vi "Cycling_No_DAQ_Tasks.vi"() -> ()   [LabVIEW 2020]
uses:
  IT-M3400/IT-M3400.lvlib
panel:
  in  "Number of Cycles":i32
  in  "Charge filepath":path
  in  "Discharge filepath":path
  in  "Batteryname":string
  in  "Starting Cycle":i32
  out "PS error out":errorcluster
  out "PS Visa Out":refnum<visa-resource-name>
  in  "Wait time":dbl
  in  "Discharge Current Setpoint":dbl format="%#.6g"
  in  "Charge Current Setpoint":dbl format="%#.6g"
  in  "Battery Type":enum16{"30Q", "40T"}(ring)
  in  "PS type":enum16{"NHR", "ITECH"}(ring)
  in  "PS error in":errorcluster caption="PS error in (no error)"
  in  "PS VISA in":refnum<visa-resource-name>
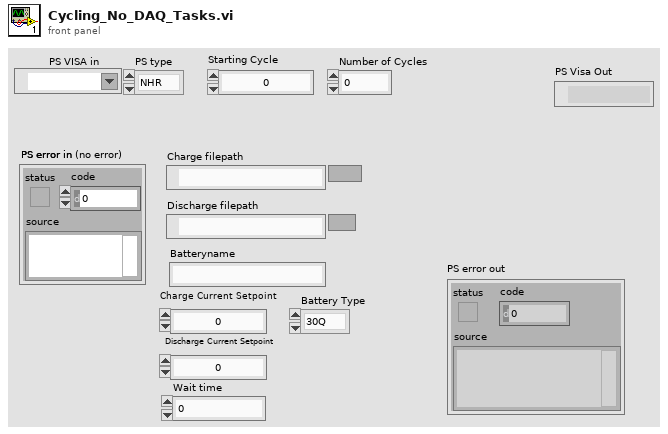
[diagram p1: front panel]
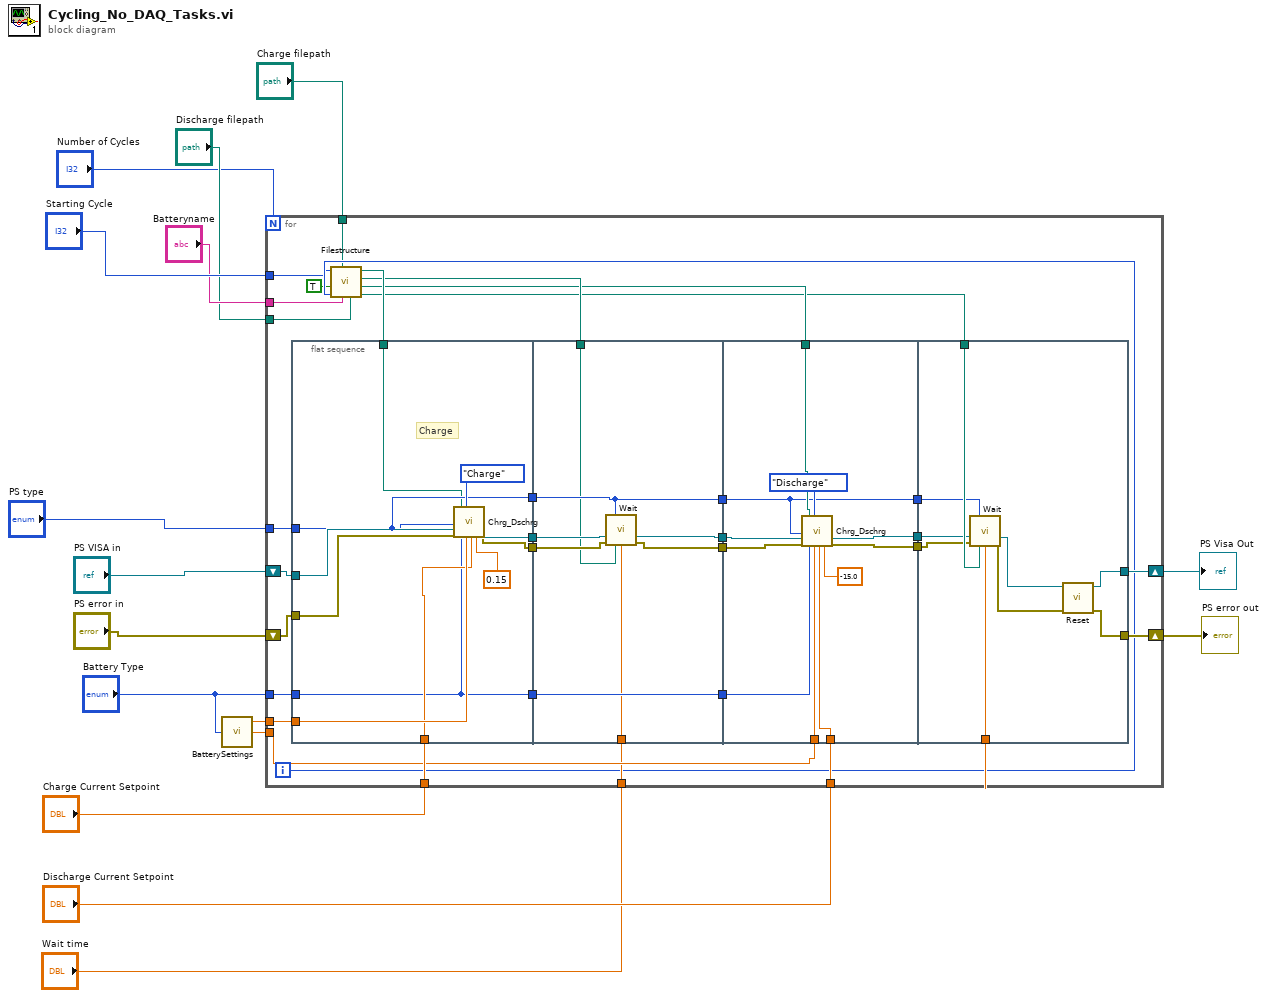
[diagram p0: block diagram]
diagram:
  n1 = call "BatterySettings.vi"("Battery Type"="Battery Type") -> ("Min Voltage (V)"=w10:dbl, "Max Voltage (V)"=w13:dbl)  [unwired: 2 in, 1 out]
  n2 = for {
    N: "Number of Cycles" -> [_]
    tunnel: "PS type" -> [w37]
    tunnel: w13 -> [w34]
    tunnel: "Battery Type" -> [w33]
    tunnel: "Charge Current Setpoint" -> [w32]
    tunnel: w10 -> [w31]
    tunnel: "Discharge Current Setpoint" -> [w30]
    tunnel: "Wait time" -> [w25]
    shift-right: [w23] -> w6
    shift-left: "PS VISA in" -> [w36]
    shift-right: [w24] -> w7
    shift-left: "PS error in" -> [w35]
    tunnel: "Starting Cycle" -> [w21]
    tunnel: "Batteryname" -> [w19]
    tunnel: "Discharge filepath" -> [w18]
    tunnel: "Charge filepath" -> [w17]
    i -> [w22]
    n3 = flat-sequence {
      tunnel: w37 -> [w51]
      tunnel: w36 -> [w59]
      tunnel: w35 -> [w58]
      tunnel: w33 -> [w50]
      tunnel: w34 -> [w55]
      tunnel: w32 -> [w54]
      tunnel: [w53] -> w48
      tunnel: [w52] -> w47
      tunnel: [w51] -> w46
      tunnel: [w50] -> w45
      tunnel: w29 -> [w49]
      tunnel: w48 -> [w67]
      tunnel: w47 -> [w66]
      tunnel: w46 -> [w63]
      tunnel: [w65] -> w44
      tunnel: [w64] -> w43
      tunnel: [w63] -> w42
      tunnel: w45 -> [w62]
      tunnel: [w62] -> w41
      tunnel: w28 -> [w61]
      tunnel: w25 -> [w60]
      tunnel: w44 -> [w78]
      tunnel: w43 -> [w77]
      tunnel: w42 -> [w68]
      tunnel: w41 -> [w76]
      tunnel: w31 -> [w75]
      tunnel: w30 -> [w74]
      tunnel: w27 -> [w71]
      tunnel: [w70] -> w40
      tunnel: [w69] -> w39
      tunnel: [w68] -> w38
      tunnel: w26 -> [w87]
      tunnel: w40 -> [w86]
      tunnel: w39 -> [w85]
      tunnel: w25 -> [w84]
      tunnel: w38 -> [w83]
      tunnel: [w79] -> w24
      tunnel: [w81] -> w23
      frame #0 {
        # "Charge"
        n4 = call "Chrg_Dschrg.vi"("PS type"=w51, "PS VISA in"=w59, "PS error in"=w58, "CyclePath"=w49, "Battery Type"=w50, "Charge/discharge"=enum8{"Charge", "Discharge"}."Charge", "Charge/Discharge Voltage Setpoint"=w55, "Current Setpoint"=w54, "Current Cutoff"=0.15) -> ("VISA resource name out"=w53:refnum<visa-resource-name>, "NHR error out"=w52:errorcluster)  [unwired: 9 in]
      }
      frame #1 {
        n5 = call "Wait.vi"("PS type"=w63, "PS VISA in"=w67, "PS error in"=w66, "Wait Filepath"=w61, "Wait time"=w60) -> ("PS Visa Out"=w65:refnum<visa-resource-name>, "PS error out"=w64:errorcluster)  [unwired: 9 in]
      }
      frame #2 {
        n6 = call "Chrg_Dschrg.vi"("PS type"=w68, "PS VISA in"=w78, "PS error in"=w77, "CyclePath"=w71, "Battery Type"=w76, "Charge/discharge"=enum8{"Charge", "Discharge"}."Discharge", "Charge/Discharge Voltage Setpoint"=w75, "Current Setpoint"=w74, "Current Cutoff"=-15.0) -> ("VISA resource name out"=w70:refnum<visa-resource-name>, "NHR error out"=w69:errorcluster)  [unwired: 9 in]
      }
      frame #3 {
        n7 = call "Wait.vi"("PS type"=w83, "PS VISA in"=w86, "PS error in"=w85, "Wait Filepath"=w87, "Wait time"=w84) -> ("PS Visa Out"=w82:refnum<visa-resource-name>, "PS error out"=w80:errorcluster)  [unwired: 9 in]
        n8 = call "Reset.vi"("error in"=w80, "VISA resource name"=w82) -> ("error out"=w79:errorcluster, "VISA resource name out"=w81:refnum<visa-resource-name>)  [unwired: 8 in]
      }
    }
    n9 = call "Filestructure.vi"("Discharge filepath"=w18, "Batteryname"=w19, "Charge filepath"=w17, "For loop i"=w22, "In for loop"=TRUE, "Starting Cycle"=w21) -> ("DischargeWaitPath"=w26:path, "DischargeCyclePath"=w27:path, "ChargeWaitPath"=w28:path, "ChargeCyclePath"=w29:path)  [unwired: 1 in, 1 out]
  }
  "PS error out" <- w7
  "PS Visa Out" <- w6
